vi "Parse Controls.vi"(8 "error in (no error)":errorcluster, 10 "VI Type":T1(ring), 11 "Controls[]":refnum<vi>[](array[refnum])) -> (0 "error out":errorcluster, 2 "Control Descriptions":string[](array[string]), 3 "Control Names":string[](array[string]))   [LabVIEW 2016]
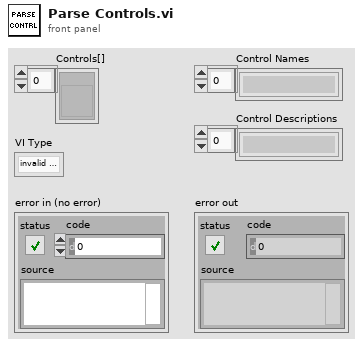
[diagram p1: front panel]
types:
  T1 = enum32{"invalid VI type", "Standard VI", "Control VI", "Global VI", "Polymorphic VI", "Configuration VI", "SubSystem", "Facade VI", "Method VI", "Statechart Diagram VI"}
  T2 = cluster{string, "result string":string, "Description out":string}
  T3 = cluster{string, "result string":string, "Description out":string}[]
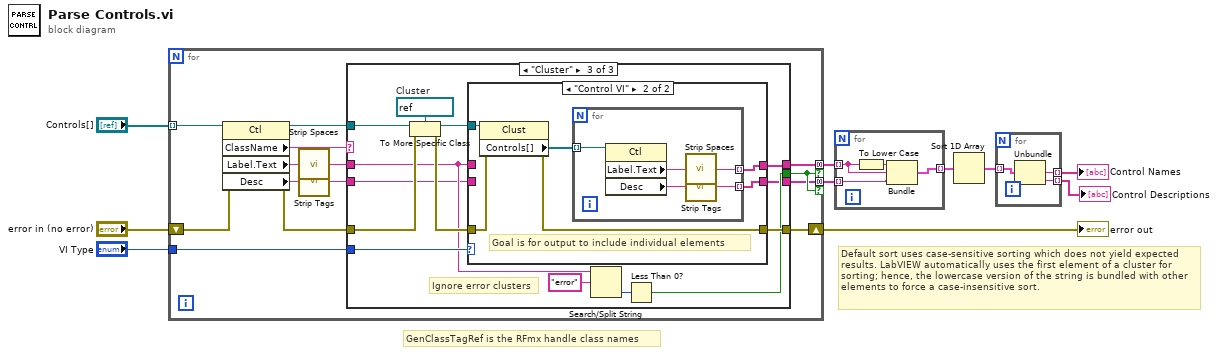
[diagram p0: block diagram]
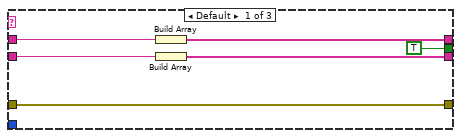
[diagram p2: hidden frame]
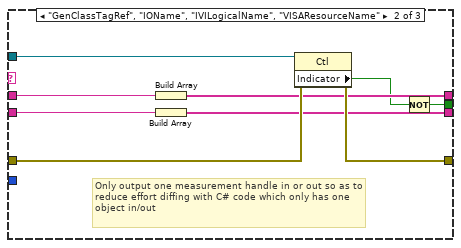
[diagram p3: hidden frame]
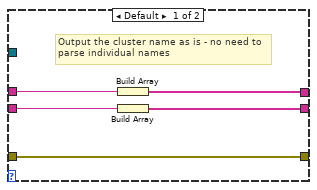
[diagram p4: hidden frame]
diagram:
  # "Default sort uses case-sensitive sorting which does not yield expected results. LabVIEW automatically uses the first element of a cluster for sorting; hence, the lowercase version of the string is bundled with other elements to force a case-insensitive sort."
  # "GenClassTagRef is the RFmx handle class names"
  n1 = for {
    tunnel: "Controls[]" -> [w23] mode=indexing
    shift-right: [w18] -> w8
    shift-left: "error in (no error)" -> [w21]
    tunnel: [w16] -> w6 mode=concatenating if=w24
    tunnel: "VI Type" -> [w15]
    tunnel: [w13] -> w2 mode=concatenating if=w24
    n2 = property class="Ctl"(reference=w23, error in=w21) -> (reference out=w22:refnum<vi>, error out=w19:errorcluster, "ClassName"=w20:string, "Label.Text"=w17:string, "Desc"=w14:string)
    n3 = call "Strip Spaces.vi"("String In"=w17) -> ("result string"=w12:string)  [unwired: 14 in]
    n4 = call "Strip Tags.vi"("Description in"=w14) -> ("Description out"=w11:string)  [unwired: 14 in]
    n5 = case shown="\"Cluster\"" w20 {
      tunnel: w22 -> [_ w35 w53]
      tunnel: w19 -> [w30 w39 w51]
      tunnel: [w30 w38 w48] -> w18
      tunnel: w12 -> [w27 w36 w42]
      tunnel: [TRUE w33 w45] -> w24
      tunnel: [w28 w37 w44] -> w16
      tunnel: w15 -> [_ _ w43]
      tunnel: w11 -> [w26 w32 w40]
      tunnel: [w25 w31 w41] -> w13
      frame Default {
        n6 = Build Array(w27) -> (w28:string[])
        n7 = Build Array(w26) -> (w25:string[])
      }
      frame "GenClassTagRef", "IOName", "IVILogicalName", "VISAResourceName" {
        # "Only output one measurement handle in or out so as to reduce effort diffing with C# code which only has one object in/out"
        n8 = Build Array(w36) -> (w37:string[])
        n9 = Build Array(w32) -> (w31:string[])
        n10 = property class="Ctl"(reference=w35, error in=w39) -> (error out=w38:errorcluster, "Indicator"=w34:bool)  [unwired: 1 out]
        n11 = Not(x=w34) -> (.not. x?=w33:bool)
      }
      frame "Cluster" {
        w50 = refnum<vi> refnum  # Cluster
        # "Ignore error clusters"
        n12 = To More Specific Class(target class=w50, reference=w53, error in=w51) -> (specific class reference=w52:refnum<vi>, error out=w49:errorcluster)
        n13 = case shown="\"Control VI\"" w43 {
          tunnel: w52 -> [_ w64]
          tunnel: w49 -> [w58 w63]
          tunnel: [w58 w62] -> w48
          tunnel: [w57 w61] -> w44
          tunnel: w42 -> [w56 _]
          tunnel: [w54 w59] -> w41
          tunnel: w40 -> [w55 _]
          frame Default {
            # "Output the cluster name as is - no need to parse individual names"
            n14 = Build Array(w56) -> (w57:string[])
            n15 = Build Array(w55) -> (w54:string[])
          }
          frame "Control VI" {
            # "Goal is for output to include individual elements"
            n16 = property class="Clust"(reference=w64, error in=w63) -> (error out=w62:errorcluster, "Controls[]"=w60:refnum<vi>[])  [unwired: 1 out]
            n17 = for {
              tunnel: w60 -> [w69] mode=indexing
              tunnel: [w67] -> w61 mode=indexing
              tunnel: [w65] -> w59 mode=indexing
              n18 = property class="Ctl"(reference=w69) -> ("Label.Text"=w68:string, "Desc"=w66:string)  [unwired: 1 in, 2 out]
              n19 = call "Strip Spaces.vi"("String In"=w68) -> ("result string"=w67:string)  [unwired: 14 in]
              n20 = call "Strip Tags.vi"("Description in"=w66) -> ("Description out"=w65:string)  [unwired: 14 in]
            }
          }
        }
        n21 = Search/Split String(string=w42, search string/char (-)="error") -> (offset of match=w46:i32)  [unwired: 1 in, 2 out]
        n22 = Less Than 0?(x=w46) -> (x < 0?=w45:bool)
      }
    }
  }
  "error out" <- w8
  n23 = for {
    tunnel: w6 -> [w73] mode=indexing
    tunnel: [w71] -> w5 mode=indexing
    tunnel: w2 -> [w70] mode=indexing
    n24 = To Lower Case(string=w73) -> (all lower case string=w72:string)
    n25 = Bundle(w72, "result string"=w73, "Description out"=w70) -> (w71:T2)  [unwired: 1 in]
  }
  n26 = Sort 1D Array(array=w5) -> (sorted array=w4:T3)
  n27 = for {
    tunnel: w4 -> [w76] mode=indexing
    tunnel: [w75] -> w3 mode=indexing
    tunnel: [w74] -> w1 mode=indexing
    n28 = Unbundle(w76) -> ("result string"=w75:string, "Description out"=w74:string)  [unwired: 1 out]
  }
  "Control Names" <- w3
  "Control Descriptions" <- w1
